vi "Initialize.vi"(8 "error in (no error)":errorcluster, 10 "config path":path, 11 "LED in":refnum<class "LED.lvclass">) -> (0 "error out":errorcluster, 3 "LED out":refnum<class "LED.lvclass">)   [LabVIEW 2016, in "LED.lvclass"]
uses:
  LED.lvclass
  LightBox/LightBox.lvclass
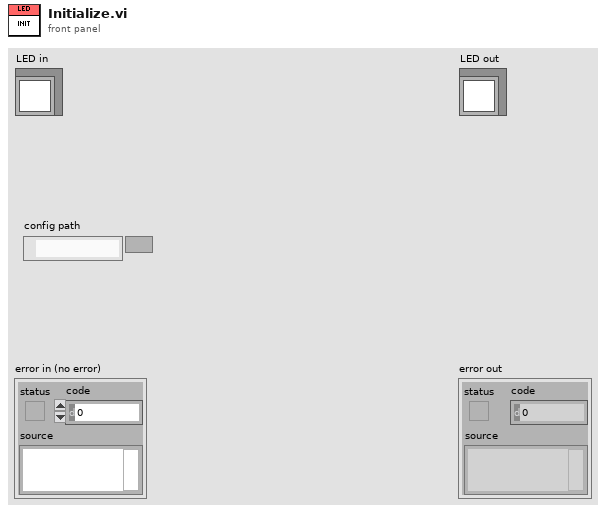
[diagram p1: front panel]
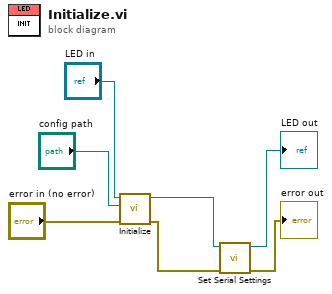
[diagram p0: block diagram]
diagram:
  n1 = call-parent "Initialize.vi"("error in (no error)"="error in (no error)", "config path"="config path", "LightBox in"="LED in") -> ("error out"=w2:errorcluster, "LightBox out"=w4:refnum<class "LED.lvclass">)  [unwired: 7 in]
  n2 = call-dynamic "Set Serial Settings.vi"("error in (no error)"=w2, "LED in"=w4) -> ("error out"=→"error out":errorcluster, "LED out"=→"LED out":refnum<class "LED.lvclass">)  [unwired: 8 in]
